vi "Testing File Reading.vi"() -> (0 "error out":errorcluster, 3 "Test result":bool)   [LabVIEW 2018, in "Config.lvlib" / "FileConfig.lvclass"]
doc: "Use this VI to test that you file is correct and there are no missing sections or unparseable sections."
uses:
  FileConfig.lvclass
  Config/Controls/Drivetrain Data.ctl
  Drive/Pod Drive/Pod.ctl
  <vilib>/Rock Robotics/WPI/ThirdParty/Phoenix-LabVIEW/Motor Controller/Controls/CTRE_Phoenix_MotorControl_SlotStructure.ctl
  Config/Controls/Elevator Data.ctl
  Config/Controls/Pneumatics Data.ctl
  <vilib>/Rock Robotics/WPI/Solenoid/WPI_SolenoidChannel.ctl
  Config/Controls/PWM Data.ctl
  <vilib>/Rock Robotics/SystemInterfaces/DIO/FPGA_DIOPWMChannel.ctl
  Config/Controls/Simulated Classes.ctl
  Drive/Pod Drive/Pod Drive.lvclass
  Config.lvclass
panel:
  out "Simulated Classes":T1
  out "File Found? 4":bool
  out "PWM Data":T2
  out "IDs found? 4":bool
  out "File Found? 3":bool
  out "Pneumatics Data":T4
  out "IDs found? 3":bool
  out "PIDFs found 2":bool
  out "File Found? 2":bool
  out "Elevator Data":T6={"Wrist"=0, "Left Master"=0, "Left Slave"=0, "Right Master"=0, "Right Slave"=0, "Elevator Wrist PID"={"P"=0.0, "I"=0.0, "D"=0.0, "F"=0.0, "integralZone"=0.0, "allowableClosedLoopError"=0, "maxIntegralAccumulator"=0.0, "closedLoopPeakOutput"=1.0, "closedLoopPeriod"=1}, "Elevator Arm PID"={"P"=0.0, "I"=0.0, "D"=0.0, "F"=0.0, "integralZone"=0.0, "allowableClosedLoopError"=0, "maxIntegralAccumulator"=0.0, "closedLoopPeakOutput"=1.0, "closedLoopPeriod"=1}, "Vacumm Pump 1"=0, "Vacumm Pump 2"=0, "Arm Motion Magic Max Velocity"=0, "Arm Motion Magic Max Acceleration"=0, "Wrist Motion Magic Max Velocity"=0, "Wrist Motion Magic Max Acceleration"=0}
  out "IDs found? 2":bool
  out "File Found?":bool
  out "PIDFs found":bool
  out "Robot Drivetrain Data":T8={"Right"={"Talon"=0, "Victor1"=0, "Victor2"=0}, "Left"={"Talon"=0, "Victor1"=0, "Victor2"=0}, "Drive Velocity Low Gear"={"P"=0.0, "I"=0.0, "D"=0.0, "F"=0.0, "integralZone"=0.0, "allowableClosedLoopError"=0, "maxIntegralAccumulator"=0.0, "closedLoopPeakOutput"=1.0, "closedLoopPeriod"=1}, "Drive Velocity High Gear"={"P"=0.0, "I"=0.0, "D"=0.0, "F"=0.0, "integralZone"=0.0, "allowableClosedLoopError"=0, "maxIntegralAccumulator"=0.0, "closedLoopPeakOutput"=1.0, "closedLoopPeriod"=1}, "Drive Motion Magic Primary Low Gear"={"P"=0.0, "I"=0.0, "D"=0.0, "F"=0.0, "integralZone"=0.0, "allowableClosedLoopError"=0, "maxIntegralAccumulator"=0.0, "closedLoopPeakOutput"=1.0, "closedLoopPeriod"=1}, "Drive Motion Magic Primary High Gear"={"P"=0.0, "I"=0.0, "D"=0.0, "F"=0.0, "integralZone"=0.0, "allowableClosedLoopError"=0, "maxIntegralAccumulator"=0.0, "closedLoopPeakOutput"=1.0, "closedLoopPeriod"=1}, "Drive Motion Magic Secondary Low Gear"={"P"=0.0, "I"=0.0, "D"=0.0, "F"=0.0, "integralZone"=0.0, "allowableClosedLoopError"=0, "maxIntegralAccumulator"=0.0, "closedLoopPeakOutput"=1.0, "closedLoopPeriod"=1}, "Drive Motion Magic Secondary High Gear"={"P"=0.0, "I"=0.0, "D"=0.0, "F"=0.0, "integralZone"=0.0, "allowableClosedLoopError"=0, "maxIntegralAccumulator"=0.0, "closedLoopPeakOutput"=1.0, "closedLoopPeriod"=1}, "Drive Right Invert"=FALSE, "Drive Right Sensor Phase"=FALSE, "Drive Left Invert"=FALSE, "Drive Left Sensor Phase"=FALSE, "Low Gear Max Velocity"=0, "High Gear Max Velocity"=0, "Motion Magic Low Gear Max Velocity"=0, "Motion Magic Low Gear Max Acceleration"=0, "Motion Magic High Gear Max Velocity"=0, "Motion Magic High Gear Max Acceleration"=0}
  out "IDs found?":bool
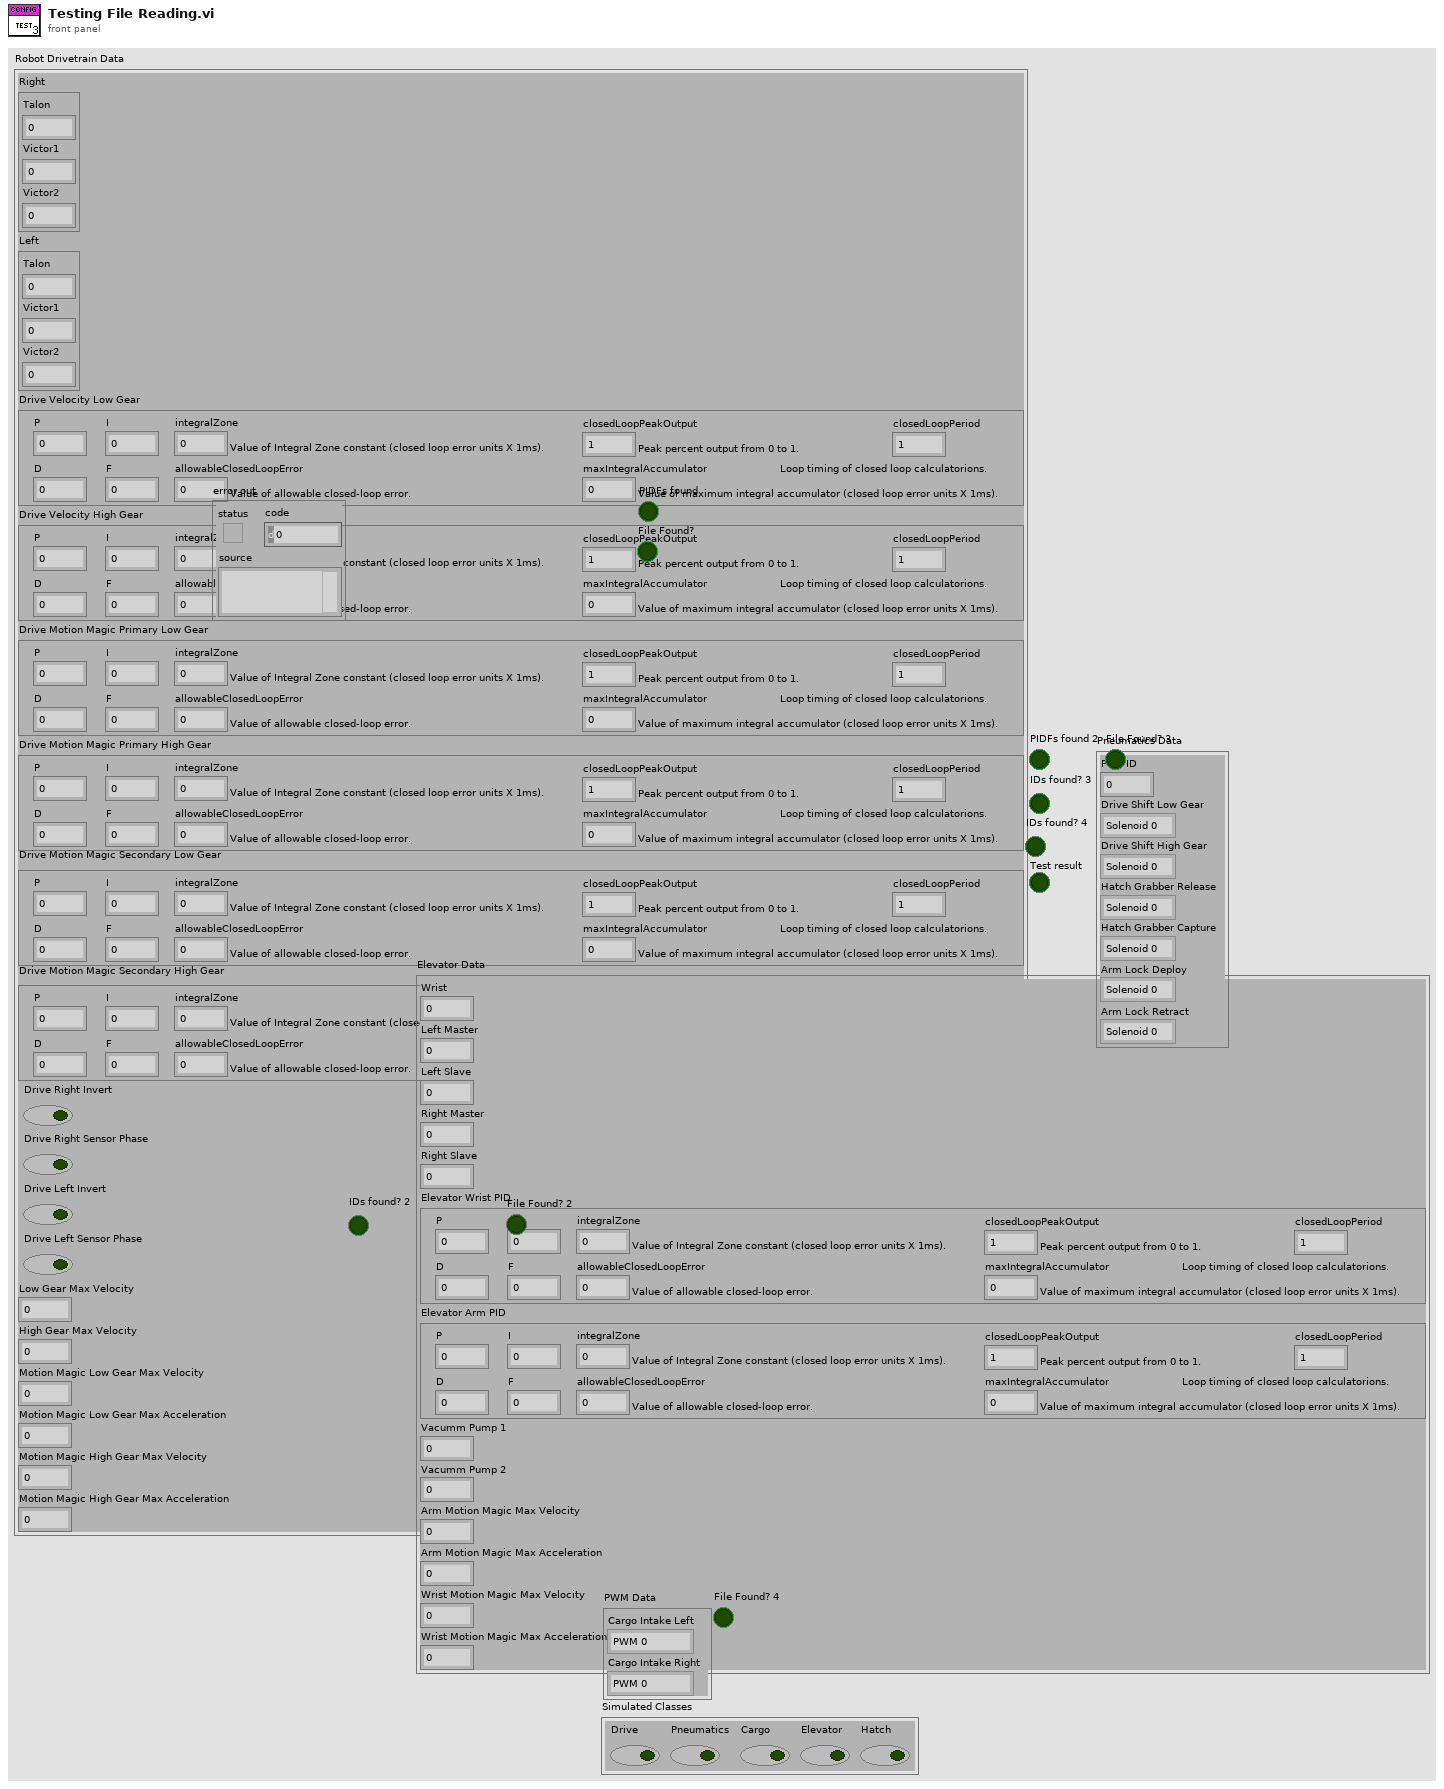
[diagram p1: front panel]
types:
  T1 = typedef "Config.lvlib/Config.lvclass/Simulated Classes.ctl" = cluster{"Drive":bool, "Pneumatics":bool, "Cargo":bool, "Elevator":bool, "Hatch":bool}
  T2 = typedef "Config.lvlib/Config.lvclass/PWM Data.ctl" = cluster{"Cargo Intake Left":T3, "Cargo Intake Right":T3}
  T3 = typedef "FPGA_DIOPWMChannel.ctl" = enum8{"PWM 0", "PWM 1", "PWM 2", "PWM 3", "PWM 4", "PWM 5", "PWM 6", "PWM 7", "PWM 8", "PWM 9", "PWM MXP 0", "PWM MXP 1", "PWM MXP 2", "PWM MXP 3", "PWM MXP 4", "PWM MXP 5", "PWM MXP 6", "PWM MXP 7", "PWM MXP 8", "PWM MXP 9", "Invalid"}
  T4 = typedef "Config.lvlib/Config.lvclass/Pneumatics Data.ctl" = cluster{"PCM ID":u8, "Drive Shift Low Gear":T5, "Drive Shift High Gear":T5, "Hatch Grabber Release":T5, "Hatch Grabber Capture":T5, "Arm Lock Deploy":T5, "Arm Lock Retract":T5}
  T5 = typedef "WPI_SolenoidChannel.ctl" = enum8{"Solenoid 0", "Solenoid 1", "Solenoid 2", "Solenoid 3", "Solenoid 4", "Solenoid 5", "Solenoid 6", "Solenoid 7", "Invalid"}
  T6 = typedef "Config.lvlib/Config.lvclass/Elevator Data.ctl" = cluster{"Wrist":u8, "Left Master":u8, "Left Slave":u8, "Right Master":u8, "Right Slave":u8, "Elevator Wrist PID":T7, "Elevator Arm PID":T7, "Vacumm Pump 1":u8, "Vacumm Pump 2":u8, "Arm Motion Magic Max Velocity":u32, "Arm Motion Magic Max Acceleration":u32, "Wrist Motion Magic Max Velocity":u32, "Wrist Motion Magic Max Acceleration":u32}
  T7 = typedef "CTRE_Phoenix_MotorControl_SlotStructure.ctl" = cluster{"P":dbl, "I":dbl, "D":dbl, "F":dbl, "integralZone":dbl, "allowableClosedLoopError":i32, "maxIntegralAccumulator":dbl, "closedLoopPeakOutput":dbl, "closedLoopPeriod":i32}
  T8 = typedef "Config.lvlib/Config.lvclass/Drivetrain Data.ctl" = cluster{"Right":T9, "Left":T9, "Drive Velocity Low Gear":T7, "Drive Velocity High Gear":T7, "Drive Motion Magic Primary Low Gear":T7, "Drive Motion Magic Primary High Gear":T7, "Drive Motion Magic Secondary Low Gear":T7, "Drive Motion Magic Secondary High Gear":T7, "Drive Right Invert":bool, "Drive Right Sensor Phase":bool, "Drive Left Invert":bool, "Drive Left Sensor Phase":bool, "Low Gear Max Velocity":u32, "High Gear Max Velocity":u32, "Motion Magic Low Gear Max Velocity":u32, "Motion Magic Low Gear Max Acceleration":u32, "Motion Magic High Gear Max Velocity":u32, "Motion Magic High Gear Max Acceleration":u32}
  T9 = typedef "Drive.lvlib/Pod Drive.lvclass/Pod.ctl" = cluster{"Talon":u8, "Victor1":u8, "Victor2":u8}
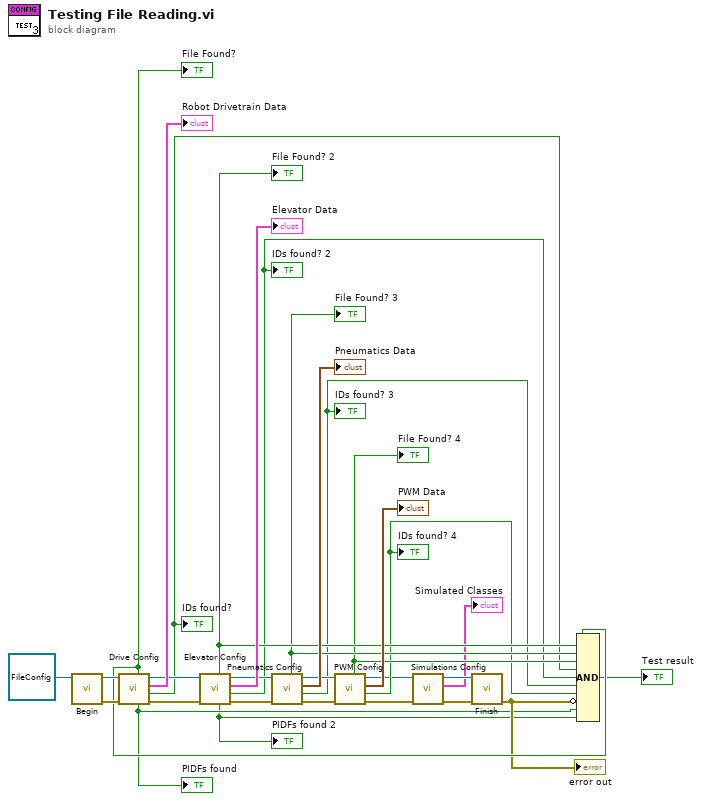
[diagram p0: block diagram]
diagram:
  n1 = call-dynamic "Begin.vi"("FileConfig in"=refnum<class "FileConfig.lvclass"> refnum ("Config.lvlib:FileConfig.lvclass")) -> ("error out"=w29:errorcluster, "FileConfig out"=w30:refnum<class "FileConfig.lvclass">)  [unwired: 8 in, 1 out]
  n2 = call-dynamic "Drive Config.vi"("error in (no error)"=w29, "FileConfig in"=w30) -> ("error out"=w28:errorcluster, "IDs found?"=w7:bool, "Robot Drivetrain Data"=→"Robot Drivetrain Data":T8, "FileConfig out"=w24:refnum<class "FileConfig.lvclass">, "PIDFs found"=w6:bool, "File Found?"=w16:bool)  [unwired: 4 in]
  "IDs found?" <- w7
  "PIDFs found" <- w6
  "File Found?" <- w16
  n3 = call-dynamic "Elevator Config.vi"("error in (no error)"=w28, "FileConfig in"=w24) -> ("error out"=w25:errorcluster, "IDs found?"=w12:bool, "Elevator Data"=→"Elevator Data":T6, "FileConfig out"=w22:refnum<class "FileConfig.lvclass">, "PIDFs found"=w5:bool, "File Found?"=w15:bool)  [unwired: 4 in]
  "IDs found? 2" <- w12
  "File Found? 2" <- w15
  "PIDFs found 2" <- w5
  n4 = call-dynamic "Pneumatics Config.vi"("error in (no error)"=w25, "FileConfig in"=w22) -> ("error out"=w19:errorcluster, "IDs found?"=w11:bool, "Pneumatics Data"=→"Pneumatics Data":T4, "FileConfig out"=w20:refnum<class "FileConfig.lvclass">, "File Found?"=w14:bool)  [unwired: 5 in]
  "IDs found? 3" <- w11
  "File Found? 3" <- w14
  n5 = call-dynamic "PWM Config.vi"("error in (no error)"=w19, "FileConfig in"=w20) -> ("error out"=w18:errorcluster, "IDs found?"=w10:bool, "PWM Data"=→"PWM Data":T2, "FileConfig out"=w3:refnum<class "FileConfig.lvclass">, "File Found?"=w13:bool)  [unwired: 5 in]
  "IDs found? 4" <- w10
  "File Found? 4" <- w13
  n6 = call-dynamic "Simulations Config.vi"("error in (no error)"=w18, "FileConfig in"=w3) -> ("error out"=w4:errorcluster, "Simulated Classes"=→"Simulated Classes":T1, "FileConfig out"=w2:refnum<class "FileConfig.lvclass">)  [unwired: 6 in, 1 out]
  n7 = call-dynamic "Finish.vi"("error in (no error)"=w4, "FileConfig in"=w2) -> ("error out"=w9:errorcluster)  [unwired: 8 in, 1 out]
  "error out" <- w9
  n8 = Compound Arithmetic op=AND(w16, w15, w14, w13, w7, w12, w11, w10, invert w9, w6, w5) -> (→"Test result":bool)
